vi "Sumadenumeros.vi"() -> ()   [LabVIEW 2022 SP3]
panel:
  in  "?":bool
  in  "Numeric 3":dbl
  out "Numeric 2":dbl
  in  "Numeric":dbl
  # "Ejercicio 1: Suma de 2 números"
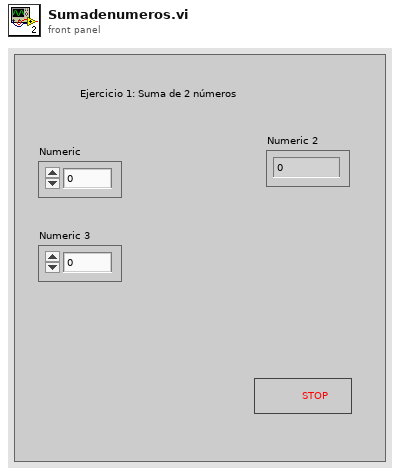
[diagram p1: front panel]
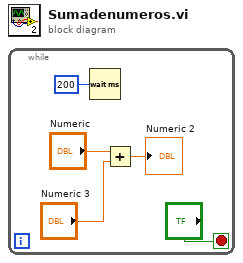
[diagram p0: block diagram]
diagram:
  n1 = while {
    stop <- "?" stop-if-true
    n2 = Wait (ms)(milliseconds to wait=u32 200 ("millisecond timer value")) -> ()  [unwired: 1 out]
    n3 = Add(x="Numeric", y="Numeric 3") -> (x+y=→"Numeric 2":dbl)
  }
